vi "Compute_Layer_Id_Patch_Permutationsvi.vi"(5 "Max_#Layers_in_a_Group":u16=2, 7 "Min_#Layers_in_a_Group":u16=2, 10 "Patch_Sizes":i32[](array[numeric])=[1, 3, 5], 11 "Layer_IDs":i32[](array[numeric])=[8, 16]) -> (3 "LayerID,PatchSize Permutations":T1[](array[typedef])=[{"[LayerID, PatchSize]"=[{"Layer_ID"=8, "Patch_Size"=1}, {"Layer_ID"=16, "Patch_Size"=1}]}, {"[LayerID, PatchSize]"=[{"Layer_ID"=8, "Patch_Size"=1}, {"Layer_ID"=16, "Patch_Size"=3}]}, {"[LayerID, PatchSize]"=[{"Layer_ID"=8, "Patch_Size"=1}, {"Layer_ID"=16, "Patch_Size"=5}]}, {"[LayerID, PatchSize]"=[{"Layer_ID"=8, "Patch_Size"=3}, {"Layer_ID"=16, "Patch_Size"=1}]}, {"[LayerID, PatchSize]"=[{"Layer_ID"=8, "Patch_Size"=3}, {"Layer_ID"=16, "Patch_Size"=3}]}, {"[LayerID, PatchSize]"=[{"Layer_ID"=8, "Patch_Size"=3}, {"Layer_ID"=16, "Patch_Size"=5}]}, {"[LayerID, PatchSize]"=[{"Layer_ID"=8, "Patch_Size"=5}, {"Layer_ID"=16, "Patch_Size"=1}]}, {"[LayerID, PatchSize]"=[{"Layer_ID"=8, "Patch_Size"=5}, {"Layer_ID"=16, "Patch_Size"=3}]}, {"[LayerID, PatchSize]"=[{"Layer_ID"=8, "Patch_Size"=5}, {"Layer_ID"=16, "Patch_Size"=5}]}])   [LabVIEW 2020]
uses:
  <vilib>/Ngene/DeepLTK Anomaly Detection Addon/Toolkit/API/Controls/Feature_Layer_Selector.ctl
  <vilib>/Ngene/DeepLTK Anomaly Detection Addon/Toolkit/DeepLTK_Anomaly_Detection_Addon.lvlib
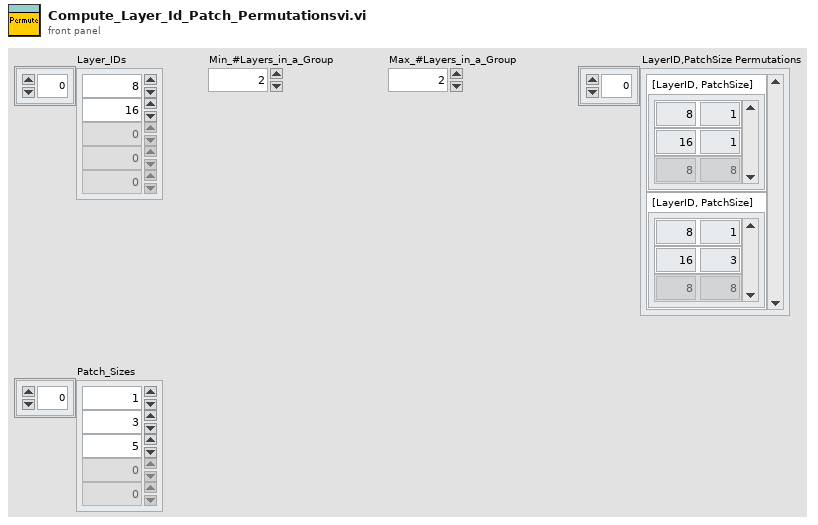
[diagram p1: front panel]
types:
  T1 = typedef "DeepLTK_Anomaly_Detection_Addon.lvlib/Feature_Layer_Selector.ctl" = cluster{"[LayerID, PatchSize]":cluster{"Layer_ID":i32, "Patch_Size":i32}[]}
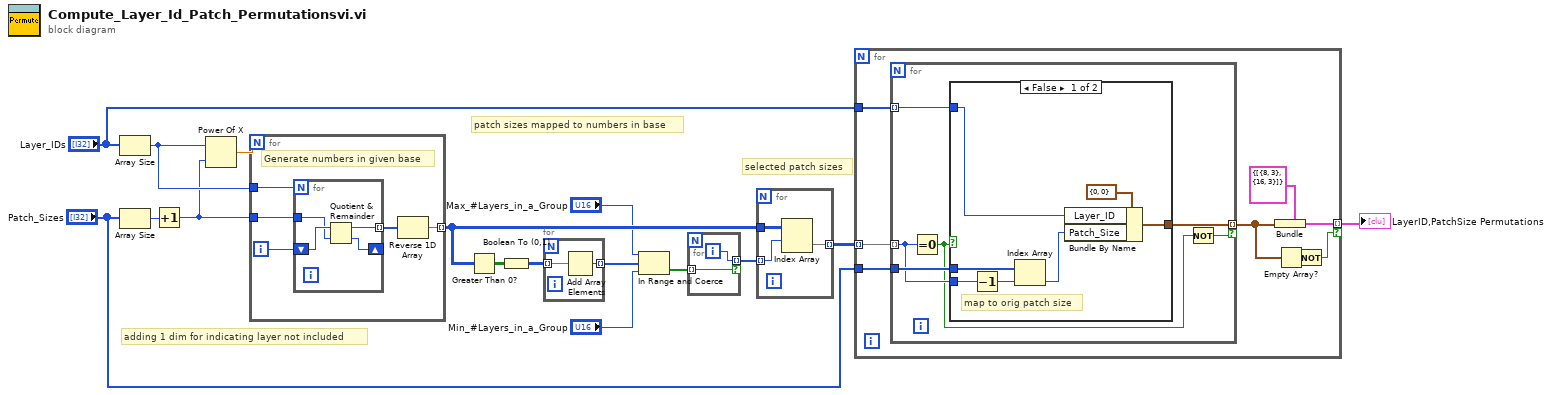
[diagram p0: block diagram]
diagram:
  # "patch sizes mapped to numbers in base"
  # "adding 1 dim for indicating layer not included"
  # "selected patch sizes"
  n1 = Array Size(array="Layer_IDs") -> (size(s)=w14:i32)
  n2 = Array Size(array="Patch_Sizes") -> (size(s)=w16:i32)
  n3 = Increment(x=w16) -> (x+1=w13:i32)
  n4 = Power Of X(1:w13, 2:w14) -> (0:w15:dbl)
  n5 = for {
    N: w15 -> [_]
    tunnel: w14 -> [w20]
    tunnel: [w18] -> w8 mode=indexing
    tunnel: w13 -> [w17]
    i -> [w21]
    # "Generate numbers in given base"
    n6 = for {
      N: w20 -> [_]
      tunnel: w17 -> [w24]
      tunnel: [w23] -> w19 mode=indexing
      shift-right: [w22] -> _
      shift-left: w21 -> [w25]
      n7 = Quotient & Remainder(x=w25, y=w24) -> (x-y*floor(x/y)=w23:i32, floor(x/y)=w22:i32)
    }
    n8 = Reverse 1D Array(array=w19) -> (reversed array=w18:i32[])
  }
  n9 = Greater Than 0?(x=w8) -> (x > 0?=w12:bool[][])
  n10 = Boolean To (0,1)(Boolean=w12) -> (0, 1=w11:i16[][])
  n11 = for {
    tunnel: w11 -> [w27] mode=indexing
    tunnel: [w26] -> w2 mode=indexing
    n12 = Add Array Elements(numeric array=w27) -> (sum=w26:i16)
  }
  n13 = In Range and Coerce(upper limit="Max_#Layers_in_a_Group", x=w2, lower limit="Min_#Layers_in_a_Group") -> (In Range?=w9:bool[])  [unwired: 1 out]
  n14 = for {
    tunnel: w9 -> [w28] mode=indexing
    tunnel: [w29] -> w7 mode=indexing if=w28
    i -> [w29]
  }
  n15 = for {
    tunnel: w8 -> [w32]
    tunnel: w7 -> [w31] mode=indexing
    tunnel: [w30] -> w6 mode=indexing
    n16 = Index Array(array=w32, index (row)=w31) -> (element=w30:i32[])  [unwired: 1 in]
  }
  n17 = for {
    tunnel: w6 -> [w40] mode=indexing
    tunnel: "Layer_IDs" -> [w39]
    tunnel: "Patch_Sizes" -> [w38]
    tunnel: [w36] -> w3 mode=indexing if=w33
    n18 = for {
      tunnel: w40 -> [w45] mode=indexing
      tunnel: w39 -> [w44] mode=indexing
      tunnel: w38 -> [w46]
      tunnel: [w43] -> w35 mode=indexing if=w41
      n19 = Equal To 0?(x=w45) -> (x = 0?=w42:bool)
      n20 = case shown="False" w42 {
        tunnel: w46 -> [w53 _]
        tunnel: w45 -> [w52 _]
        tunnel: w44 -> [w50 _]
        tunnel: [w48 _] -> w43
        frame False {
          # "map to orig patch size"
          n21 = Decrement(x=w52) -> (x-1=w47:i32)
          n22 = Index Array(array=w53, index=w47) -> (element=w49:i32)
          n23 = Bundle By Name(cluster=cluster{"Layer_ID":i32, "Patch_Size":i32} {"Layer_ID"=0, "Patch_Size"=0} ("Cluster"), "Layer_ID"=w50, "Patch_Size"=w49) -> (w48:cluster{"Layer_ID":i32, "Patch_Size":i32})
        }
        frame True {
          # "skip"
        }
      }
      n24 = Not(x=w42) -> (.not. x?=w41:bool)
    }
    n25 = Bundle(cluster=T1 {"[LayerID, PatchSize]"=[{"Layer_ID"=8, "Patch_Size"=3}, {"Layer_ID"=16, "Patch_Size"=3}]} ("Feature_Layers 2"), "[LayerID, PatchSize]"=w35) -> (w36:T1)
    n26 = Empty Array?(array=w35) -> (empty?=w34:bool)
    n27 = Not(x=w34) -> (.not. x?=w33:bool)
  }
  "LayerID,PatchSize Permutations" <- w3
